vi "Init_Action.vi"(8 "error in":errorcluster caption="错误输入（无错误）", 11 "AutoDetPort":bool) -> (0 "error out":errorcluster caption="错误输出")   [LabVIEW 2013]
uses:
  GlobValue.vi
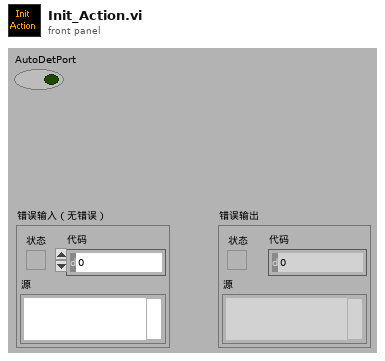
[diagram p1: front panel]
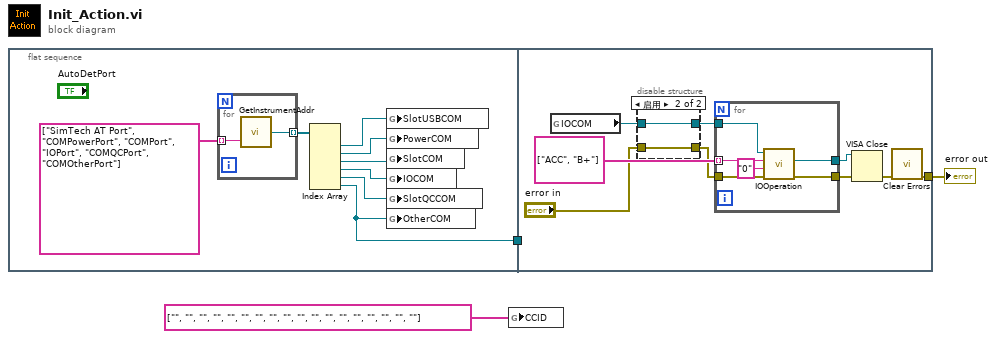
[diagram p0: block diagram]
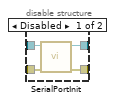
[diagram p2: hidden frame]
diagram:
  n1 = flat-sequence {
    tunnel: [w4] -> w2
    tunnel: [w14] -> w3
    tunnel: w2 -> [_]
    frame #0 {
      n2 = for {
        tunnel: string[] ["SimTech AT Port", "COMPowerPort", "COMPort", "IOPort", "COMQCPort", "COMOtherPort"] ("数组") -> [w13] mode=indexing
        tunnel: [w12] -> w10 mode=indexing
        n3 = call "GetInstrumentAddr.vi"("String"=w13) -> ("VISA session"=w12:refnum<visa-resource-name>)  [unwired: 1 out]
      }
      n4 = Index Array(array=w10) -> (element #1=w9:refnum<visa-resource-name>, element #2=w8:refnum<visa-resource-name>, element #3=w7:refnum<visa-resource-name>, element #4=w6:refnum<visa-resource-name>, element #5=w5:refnum<visa-resource-name>, element #6=w4:refnum<visa-resource-name>)  [unwired: 6 in]
      n5 = global write "GlobValue.vi" "SlotUSBCOM"(w9) -> ()
      n6 = global write "GlobValue.vi" "PowerCOM"(w8) -> ()
      n7 = global write "GlobValue.vi" "SlotCOM"(w7) -> ()
      n8 = global write "GlobValue.vi" "IOCOM"(w6) -> ()
      n9 = global write "GlobValue.vi" "SlotQCCOM"(w5) -> ()
      n10 = global write "GlobValue.vi" "OtherCOM"(w4) -> ()
    }
    frame #1 {
      n11 = global read "GlobValue.vi" "IOCOM"() -> (w21:refnum<visa-resource-name>)
      n12 = disable-structure shown="启用" {
        disable-tunnel: w21 -> [w26 w28]
        disable-tunnel: [w25 w28] -> w20
        disable-tunnel: "error in" -> [w24 w27]
        disable-tunnel: [w23 w27] -> w18
        frame Disabled {
          n13 = call "SerialPortInit.vi"("错误输入"=w24, "COMIn"=w26) -> ("错误输出"=w23:errorcluster, "COMOut"=w25:refnum<visa-resource-name>)  [unwired: 8 in]
        }
        frame Enabled {
        }
      }
      n14 = for "For循环" {
        tunnel: string[] ["ACC", "B+"] -> [w34] mode=indexing
        tunnel: w20 -> [w33]
        tunnel: w18 -> [w31]
        tunnel: [w30] -> w17
        tunnel: [w29] -> w16
        n15 = call "IOOperation.vi"("error in"=w31, "Value"="0", "Channel"=w34, "Com"=w33) -> ("error out"=w30:errorcluster, "ComOut"=w29:refnum<visa-resource-name>)  [unwired: 5 in, 1 out]
      }
      n16 = VISA Close(VISA resource name=w16, error in (no error)=w17) -> (error out=w15:errorcluster)
      n17 = call <vilib>:"Clear Errors.vi"("error in (no error)"=w15) -> ("error out"=w14:errorcluster)  [unwired: 6 in]
    }
  }
  n18 = global write "GlobValue.vi" "CCID"(string[] ["", "", "", "", "", "", "", "", "", "", "", "", "", "", "", "", "", ""] ("CCID")) -> ()
  "error out" <- w3
